vi "SinglePointMeasurement2450.vi"(7 "error out 2":errorcluster, 8 "Measure":T1, 10 "VISA resource name 2":refnum<visa-resource-name>) -> (0 "error out":errorcluster, 1 "String":string, 2 "reading":string, 3 "VISA resource name":refnum<visa-resource-name>, 4 "Measuremet":dbl)   [LabVIEW 2021]
uses:
  Measure2450.ctl
panel:
  out "x-y":u32
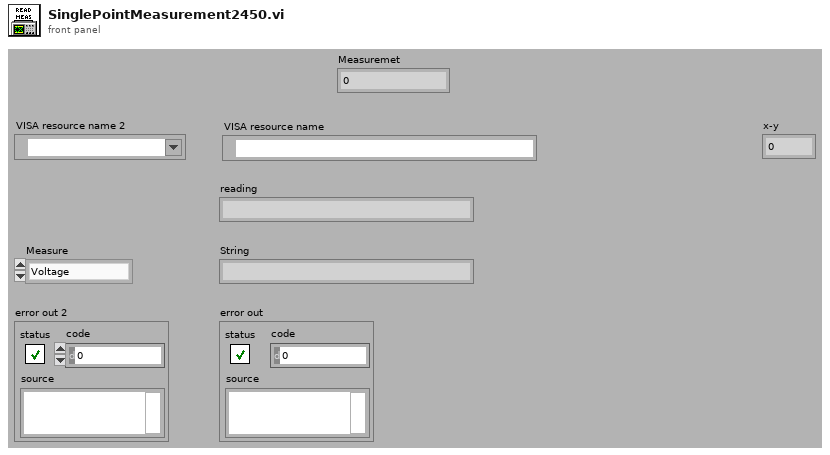
[diagram p1: front panel]
types:
  T1 = typedef "Measure2450.ctl" = enum16{"Voltage", "Current"}
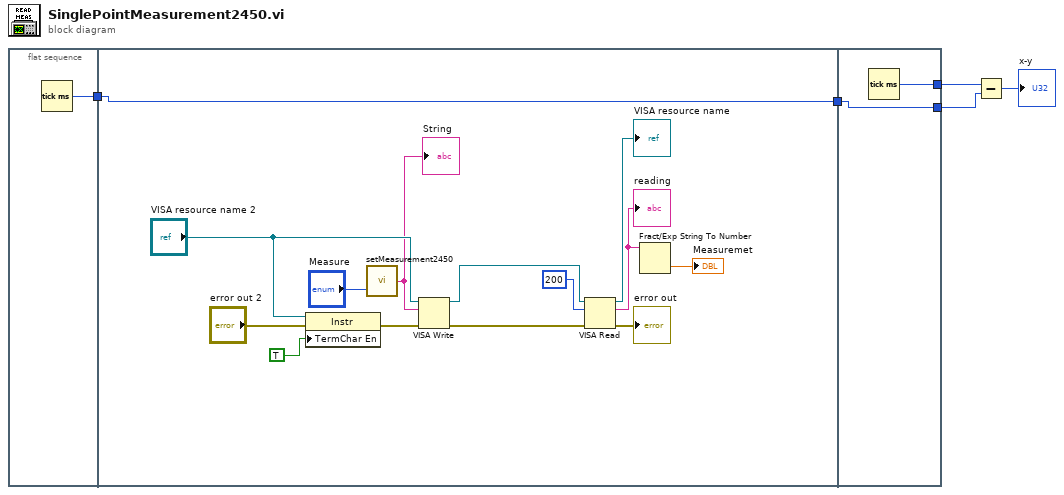
[diagram p0: block diagram]
diagram:
  n1 = flat-sequence {
    tunnel: [w6] -> w5
    tunnel: w5 -> [w8]
    tunnel: [w8] -> w4
    tunnel: w4 -> [w21]
    tunnel: [w22] -> w3
    tunnel: [w21] -> w2
    frame #0 {
      n2 = Tick Count (ms)() -> (millisecond timer value=w6:u32)
    }
    frame #1 {
      n3 = property class="Instr"(reference="VISA resource name 2", error in="error out 2", "TermChar En"=TRUE ("Message Based Settings:Termination Character Enable")) -> (error out=w11:errorcluster)  [unwired: 1 out]
      n4 = call "setMeasurement2450.vi"("Measure"="Measure") -> ("String"=w9:string)  [unwired: 1 in]
      "String" <- w9
      n5 = VISA Write(VISA resource name="VISA resource name 2", write buffer=w9, error in (no error)=w11) -> (VISA resource name out=w18:refnum<visa-resource-name>, error out=w7:errorcluster)  [unwired: 1 out]
      n6 = VISA Read(VISA resource name=w18, byte count=u32 200, error in (no error)=w7) -> (VISA resource name out=→"VISA resource name":refnum<visa-resource-name>, read buffer=w15:string, error out=→"error out":errorcluster)  [unwired: 1 out]
      "reading" <- w15
      n7 = Fract/Exp String To Number(string=w15) -> (number=→"Measuremet":dbl)  [unwired: 3 in, 1 out]
    }
    frame #2 {
      n8 = Tick Count (ms)() -> (millisecond timer value=w22:u32)
    }
  }
  n9 = Subtract(x=w3, y=w2) -> (x-y=→"x-y":u32)
